vi "DblMonoPMDScan.vi"() -> ()   [LabVIEW 2009]
uses:
  <vilib>/Utility/file.llb/Write To Spreadsheet File (DBL).vi
  <vilib>/Analysis/NI_AALBase.lvlib
panel:
  in  "On":bool=TRUE
  out "Power":cluster{dbl[], dbl[]}(graph)
  out "Waveform Chart":dbl(graph)
  in  "Save":bool=TRUE
  in  "Scan Save Path":path
  in  "Exit":bool
  in  "STOP":bool
  in  "Step Time (sec)":dbl=1.0 min=0.001 max=300.0 step=0.001 format="%.3f"
  in  "Step Size (nm)":dbl=1.0 min=0.1 max=100.0 step=0.1 format="%.1f"
  in  "End":dbl=800.0 min=0.0 max=2000.0 step=0.1 format="%.1f"
  in  "Start":dbl=400.0 min=0.0 max=2000.0 step=0.1 format="%.1f"
  in  "Scan":bool
  in  "Up":bool=TRUE caption="Down"
  in  "Increment (nm)":dbl=10.0 min=0.1 max=2000.0 step=0.1 format="%.1f"
  in  "PMD Settings":T1={"Beam Diameter (mm)"=4.0, "BWIn"=0, "Averaging Rate"=300, "Auto Range"=TRUE} {"Averaging Rate" min=33 max=5000 step=1; "BWIn" items=["HIGH", "LOW"]; "Beam Diameter (mm)" min=1.0 max=9.0 step=0.5}
  in  "Step":bool
  out "Busy":bool
  in  "Send Command":bool
  in  "Command":u16(ring) items=["nm", "goto", "nm/min", "VIS grating", "IR grating"]
  in  "Wavelength (nm)":dbl=100.0 min=0.0 max=2000.0 step=0.1 format="%.1f"
  in  "Scan Speed (nm/min)":dbl=100.0 min=1.0 max=500.0 step=0.1 format="%.1f"
  out "Done?":string
  in  "Send Question":bool
  in  "Ask?":u16(ring) items=["?nm", "?nm/min", "?grating", "?turret", "?gratings"]
  out "Power (W)":dbl format="%^#_9e"
  in  "Zero?":bool
  out "PM Error log":string
  out "AUTO?":bool
  out "Zero Value":dbl format="%#.3p"
  out "Rng":string
  in  "Range":i16=1 min=1 max=6 step=1
  in  "Mono Port":refnum<visa-resource-name>="COM5"
  out "IDN String":string
  out "Sensor SN":string
  out "Sensor Name":string
  out "Reply":string caption="Mono Response"
  # "Range Settings"
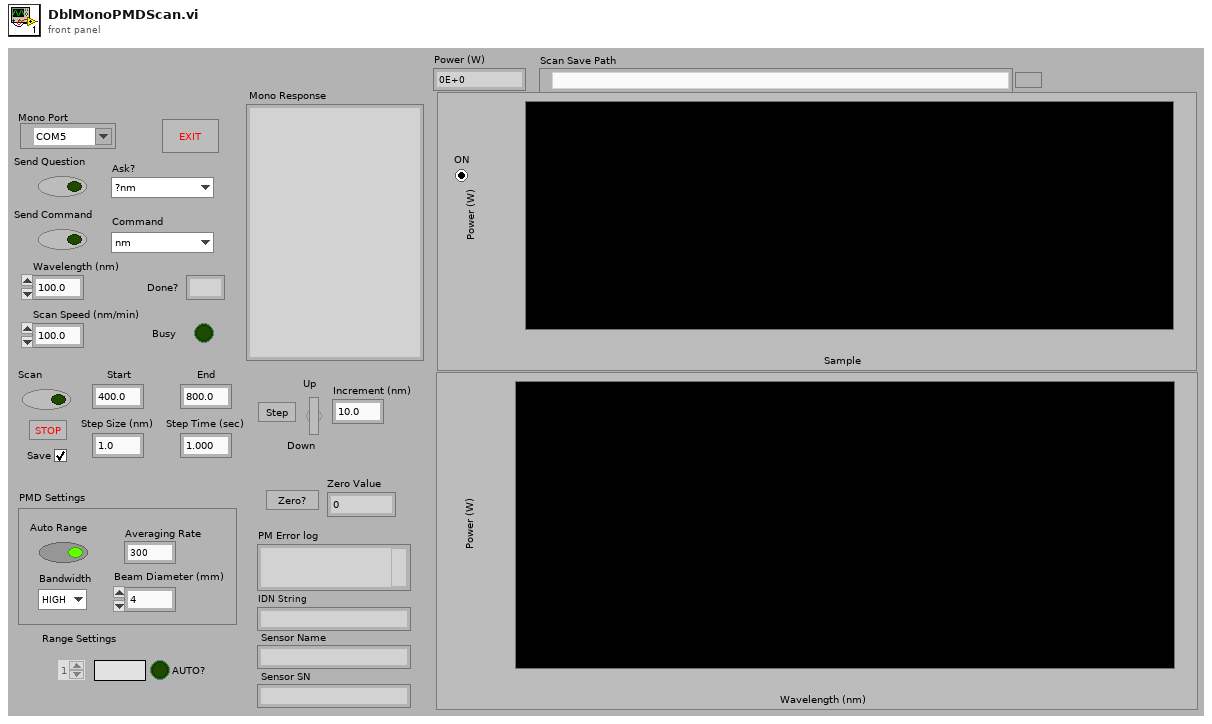
[diagram p1: front panel]
types:
  T1 = cluster{"Beam Diameter (mm)":dbl, "BWIn":u16, "Averaging Rate":i32, "Auto Range":bool}
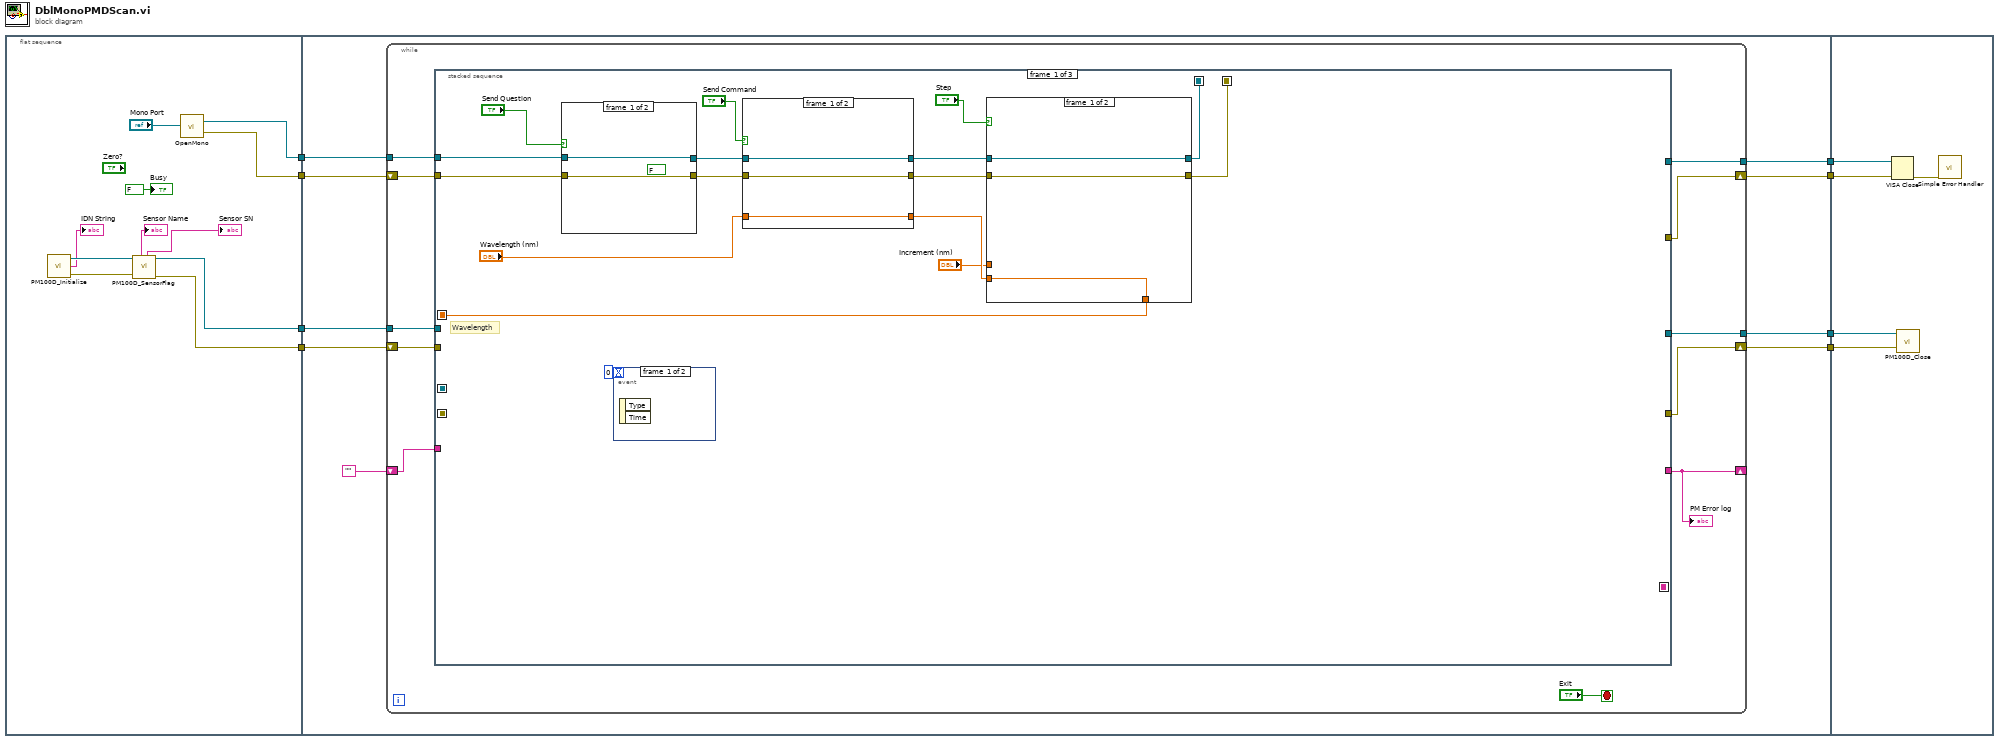
[diagram p0: block diagram]
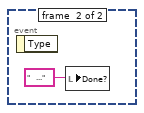
[diagram p2: hidden frame]
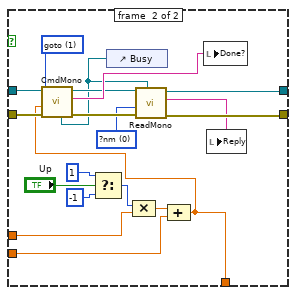
[diagram p3: hidden frame]
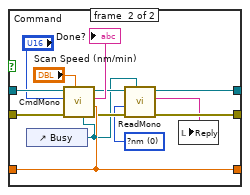
[diagram p4: hidden frame]
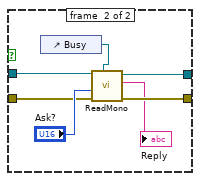
[diagram p5: hidden frame]
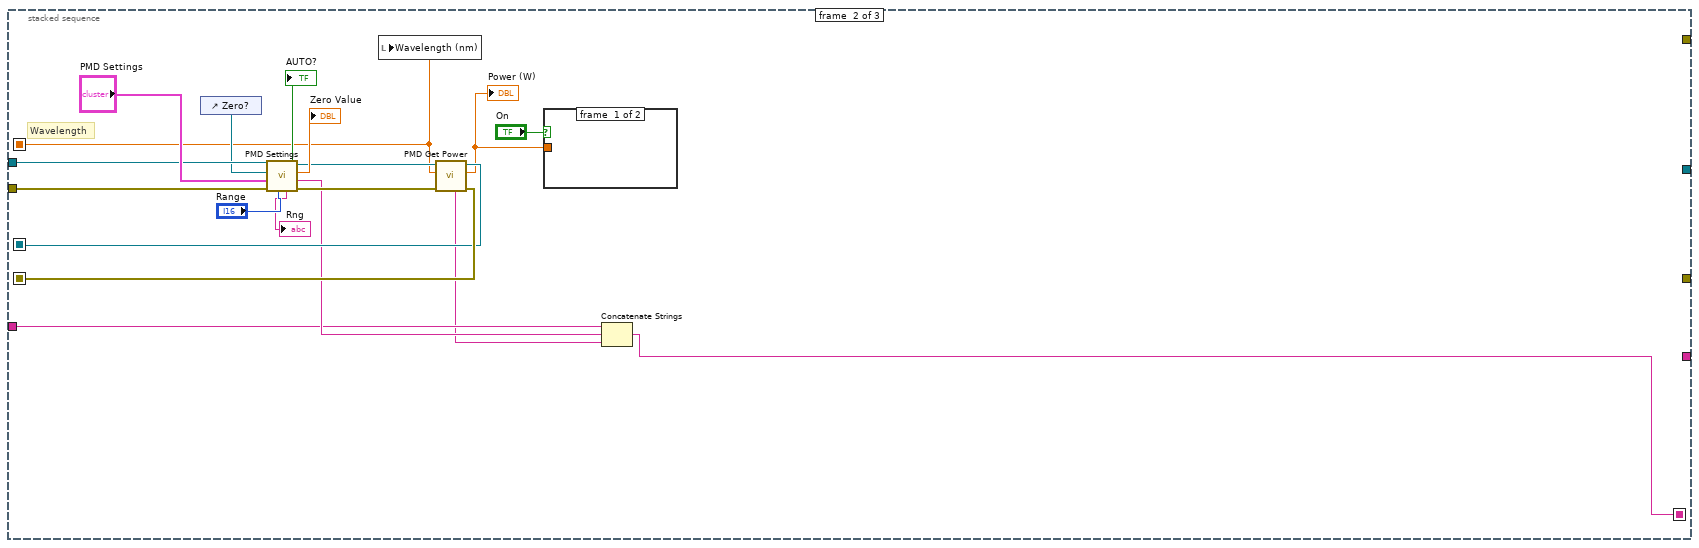
[diagram p6: hidden frame]
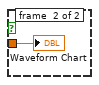
[diagram p7: hidden frame]
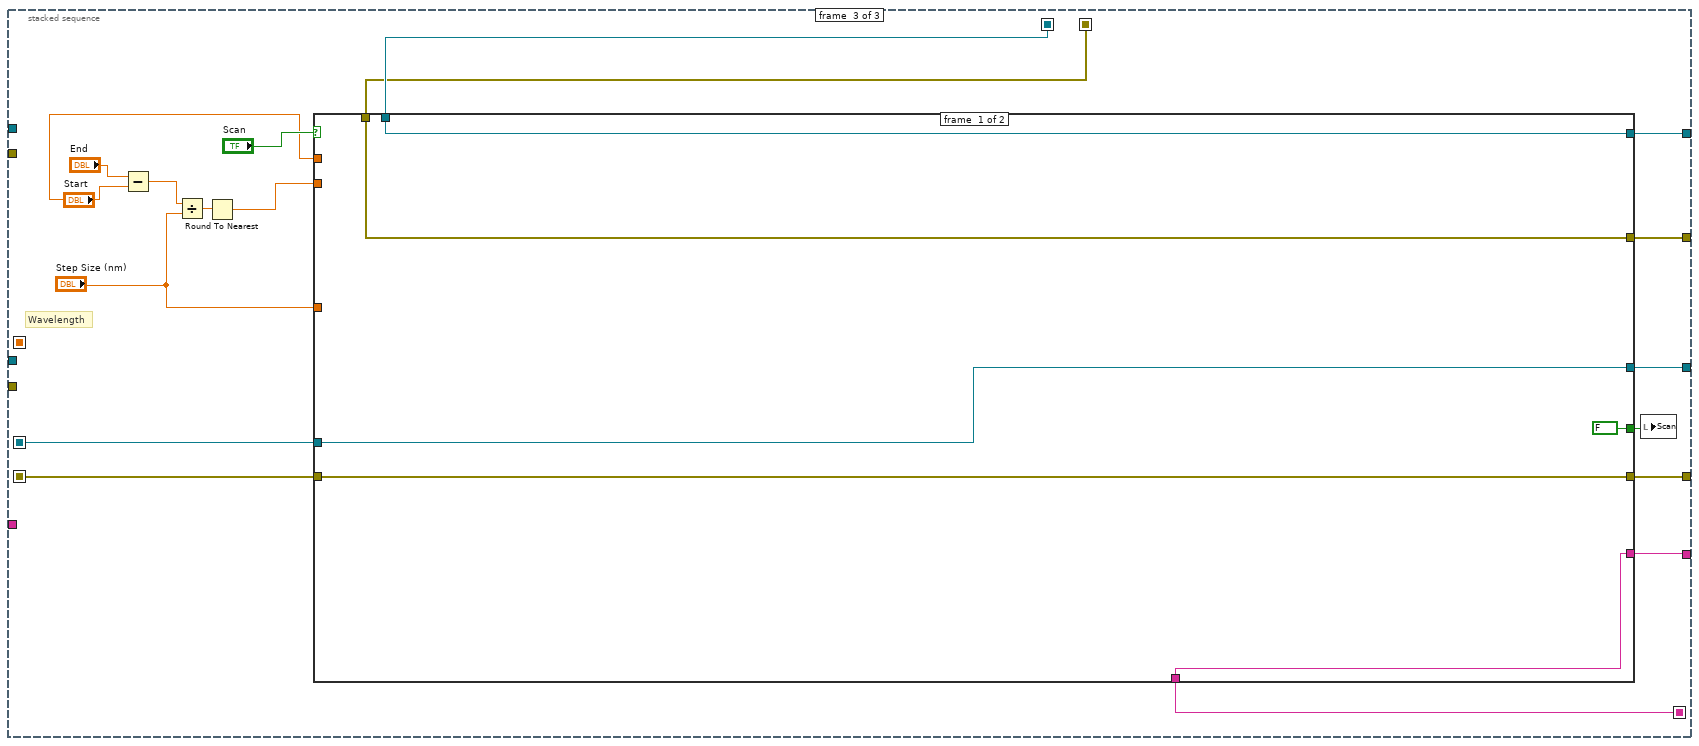
[diagram p8: hidden frame]
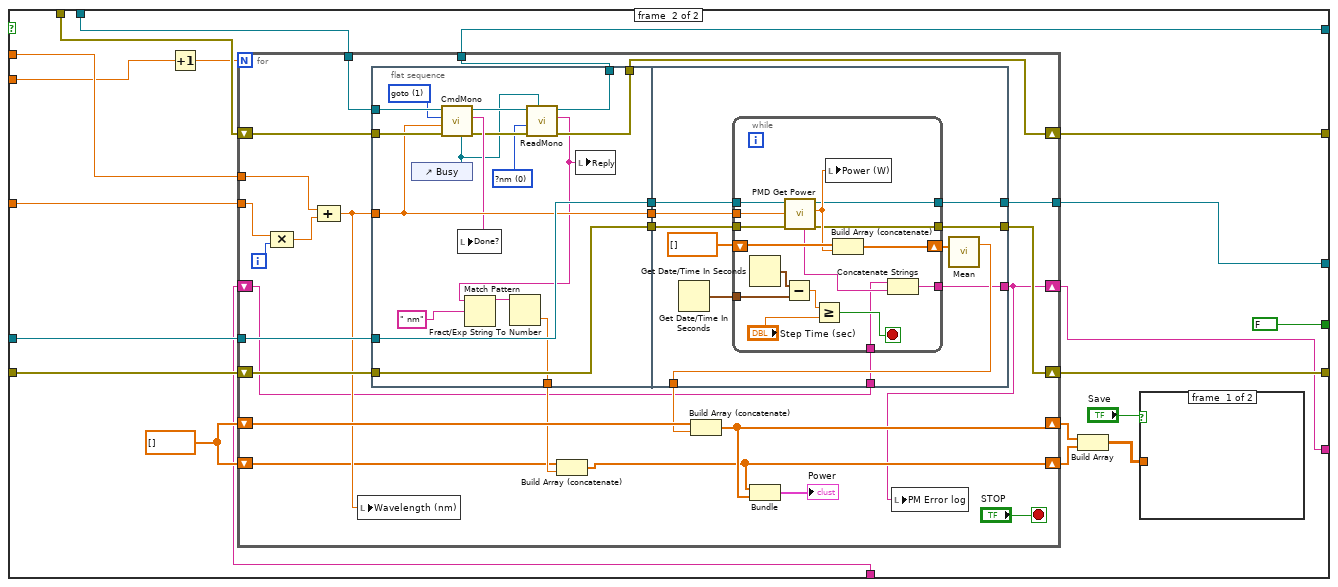
[diagram p9: hidden frame]
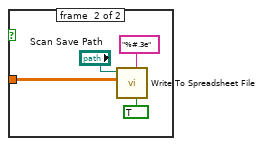
[diagram p10: hidden frame]
diagram:
  n1 = flat-sequence {
    tunnel: [w14] -> w8
    tunnel: [w13] -> w7
    tunnel: [w12] -> w6
    tunnel: [w11] -> w5
    tunnel: w8 -> [w27]
    tunnel: w7 -> [w28]
    tunnel: w6 -> [w26]
    tunnel: w5 -> [w25]
    tunnel: [w24] -> w4
    tunnel: [w23] -> w3
    tunnel: [w22] -> w2
    tunnel: [w21] -> w1
    tunnel: w4 -> [w245]
    tunnel: w3 -> [w244]
    tunnel: w2 -> [w243]
    tunnel: w1 -> [w242]
    frame #0 {
      n2 = call "PM100D_Initialize.vi"() -> ("error out"=w18:errorcluster, "Instrument"=→"IDN String":string, "VISA out"=w19:refnum<visa-resource-name>)  [unwired: 2 in, 1 out]
      n3 = call "PM100D_SensorFlag.vi"("error in (no error)"=w18, "VISA in"=w19) -> ("error out"=w14:errorcluster, "VISA out"=w13:refnum<visa-resource-name>, "sn"=→"Sensor SN":string, "name"=→"Sensor Name":string)  [unwired: 2 in, 4 out]
      n4 = call "OpenMono.vi"("Mono Port"="Mono Port") -> ("VISA resource name out"=w12:refnum<visa-resource-name>, "error out"=w11:errorcluster)
      "Busy" <- FALSE ("Busy")
    }
    frame #1 {
      n5 = while {
        tunnel: w28 -> [w37]
        tunnel: w26 -> [w39]
        tunnel: [w34] -> w23
        tunnel: [w32] -> w21
        shift-right: [w31] -> w22
        shift-left: w27 -> [w36]
        shift-right: [w33] -> w24
        shift-left: w25 -> [w38]
        shift-right: [w29] -> _
        shift-left: "" -> [w30]
        stop <- "Exit" stop-if-true
        n6 = stacked-sequence {
          seq-local: [w40 _ _] -> [_ w104 _]
          seq-local: [w45 _ _] -> [_ _ w134]
          seq-local: [w44 _ _] -> [_ _ w133]
          seq-local: [_ w112 _] -> [_ _ w132]
          seq-local: [_ w113 _] -> [_ _ w131]
          seq-local: [_ w105 _] -> [_ _ w125]
          tunnel: w39 -> [w51 _ _]
          tunnel: w38 -> [w50 _ _]
          tunnel: w37 -> [_ w115 _]
          tunnel: w36 -> [_ w114 _]
          tunnel: [_ _ w130] -> w34
          tunnel: [_ _ w129] -> w33
          tunnel: [_ _ w128] -> w32
          tunnel: [_ _ w127] -> w31
          tunnel: w30 -> [_ w107 _]
          tunnel: [_ _ w124] -> w29
          frame #0 {
            # "Wavelength"
            n7 = case shown="True" "Send Question" {
              tunnel: w51 -> [w96 w102]
              tunnel: w50 -> [w95 w101]
              tunnel: [w96 w100] -> w53
              tunnel: [w95 w99] -> w52
              frame #0 {
                (unwired) FALSE ("Read Error")
              }
              frame #1 {
                n8 = control-ref of="Busy"() -> (w97:refnum<vi>)
                n9 = call "ReadMono.vi"("Busy"=w97, "error in (no error)"=w101, "Cmd"="Ask?", "Mono Port"=w102) -> ("error out"=w99:errorcluster, "Response"=→"Reply":string, "Mono Port Out"=w100:refnum<visa-resource-name>)  [unwired: 2 in, 1 out]
              }
            }
            n10 = event shown="[1] \"Send Command\", \"Step\": Mouse Up" {
              selector: _ -> [_ _]
              dyn-events: _ -> [_ _]
              timeout: 0 -> [_ _]
              event #0 {
                n11 = event-data() -> ()  [unwired: 1 in, 2 out]
              }
              event #1 {
                n12 = event-data() -> ()  [unwired: 1 in, 1 out]
                n13 = local write "Done?"("   ..." ("Done?")) -> ()
              }
            }
            n14 = case shown="True" "Send Command" {
              tunnel: w53 -> [w81 w94]
              tunnel: w52 -> [w80 w93]
              tunnel: [w81 w86] -> w48
              tunnel: [w80 w85] -> w47
              tunnel: "Wavelength (nm)" -> [w79 w89]
              tunnel: [w79 w89] -> w46
              frame #0 {
              }
              frame #1 {
                w84 = u16 0 items=["?nm", "?nm/min", "?grating", "?turret", "?gratings"] ("Cmd")
                n15 = control-ref of="Busy"() -> (w82:refnum<vi>)
                n16 = call "CmdMono.vi"("Busy"=w82, "Scan Speed (nm/min)"="Scan Speed (nm/min)", "error in (no error)"=w93, "Wavelength (nm)"=w89, "Cmd"="Command", "Mono Port"=w94) -> ("error out"=w87:errorcluster, "Response"=→"Done?":string, "Mono Port Out"=w88:refnum<visa-resource-name>)  [unwired: 2 in, 1 out]
                n17 = call "ReadMono.vi"("Busy"=w82, "error in (no error)"=w87, "Cmd"=w84, "Mono Port"=w88) -> ("error out"=w85:errorcluster, "Response"=w83:string, "Mono Port Out"=w86:refnum<visa-resource-name>)  [unwired: 2 in, 1 out]
                n18 = local write "Reply"(w83) -> ()
              }
            }
            n19 = case shown="True" "Step" {
              tunnel: w48 -> [w59 w78]
              tunnel: w47 -> [w58 w77]
              tunnel: w46 -> [w57 w71]
              tunnel: [w59 w64] -> w45
              tunnel: [w58 w65] -> w44
              tunnel: "Increment (nm)" -> [_ w70]
              tunnel: [w57 w60] -> w40
              frame #0 {
              }
              frame #1 {
                w62 = u16 0 items=["?nm", "?nm/min", "?grating", "?turret", "?gratings"] ("Cmd")
                w69 = u16 1 items=["nm", "goto", "nm/min", "VIS grating", "IR grating"] ("Cmd")
                n20 = Select(t=1, s="Up", f=-1) -> (s? t:f=w76:i32)
                n21 = control-ref of="Busy"() -> (w61:refnum<vi>)
                n22 = Compound Arithmetic op=MULTIPLY(w76, w70) -> (w72:dbl)
                n23 = Compound Arithmetic op=ADD(w72, w71) -> (w60:dbl)
                n24 = call "CmdMono.vi"("Busy"=w61, "error in (no error)"=w77, "Wavelength (nm)"=w60, "Cmd"=w69, "Mono Port"=w78) -> ("error out"=w66:errorcluster, "Response"=w68:string, "Mono Port Out"=w67:refnum<visa-resource-name>)  [unwired: 3 in, 1 out]
                n25 = call "ReadMono.vi"("Busy"=w61, "error in (no error)"=w66, "Cmd"=w62, "Mono Port"=w67) -> ("error out"=w65:errorcluster, "Response"=w63:string, "Mono Port Out"=w64:refnum<visa-resource-name>)  [unwired: 2 in, 1 out]
                n26 = local write "Done?"(w68) -> ()
                n27 = local write "Reply"(w63) -> ()
              }
            }
          }
          frame #1 {
            # "Wavelength"
            n28 = control-ref of="Zero?"() -> (w109:refnum<vi>)
            n29 = call "PMD Settings.vi"("Visa In"=w115, "Zero?"=w109, "PMD Settings In"="PMD Settings", "Error In"=w114, "Range"="Range") -> ("AUTO?"=→"AUTO?":bool, "Rng"=→"Rng":string, "Visa Out"=w118:refnum<visa-resource-name>, "ZeroValue"=→"Zero Value":dbl, "PM Error log"=w108:string, "error out"=w117:errorcluster)
            n30 = local write "Wavelength (nm)"(w104) -> ()
            n31 = call "PMD Get Power.vi"("VISA In"=w118, "Wavelength (nm)"=w104, "error in"=w117) -> ("PMD Error"=w106:string, "VISA out"=w112:refnum<visa-resource-name>, "Readout value"=w111:dbl, "error out"=w113:errorcluster)  [unwired: 1 in, 2 out]
            "Power (W)" <- w111
            n32 = case shown="True" "On" {
              tunnel: w111 -> [_ w123]
              frame #0 {
              }
              frame #1 {
                "Waveform Chart" <- w123
              }
            }
            n33 = Concatenate Strings(w107, w108, w106) -> (w105:string)
          }
          frame #2 {
            # "Wavelength"
            n34 = Subtract(x="End", y="Start") -> (x-y=w139:dbl)
            n35 = Divide(x=w139, y="Step Size (nm)") -> (x/y=w138:dbl)
            n36 = Round To Nearest(number=w138) -> (nearest integer value=w137:dbl)
            n37 = case shown="True" "Scan" {
              tunnel: w137 -> [_ w162]
              tunnel: w133 -> [w145 w164]
              tunnel: w134 -> [w144 w165]
              tunnel: "Start" -> [_ w167]
              tunnel: "Step Size (nm)" -> [_ w166]
              tunnel: w132 -> [w147 w160]
              tunnel: w131 -> [w146 w159]
              tunnel: [w147 w157] -> w128
              tunnel: [w146 w158] -> w127
              tunnel: [w145 w156] -> w129
              tunnel: [w144 w155] -> w130
              tunnel: [FALSE ("Scan") FALSE ("Scan")] -> w126
              tunnel: w125 -> [w142 w149]
              tunnel: [w142 w148] -> w124
              frame #0 {
              }
              frame #1 {
                w163 = dbl[] []
                n38 = Increment(x=w162) -> (x+1=w161:dbl)
                n39 = for {
                  N: w161 -> [_]
                  tunnel: w165 -> [w194]
                  tunnel: w167 -> [w190]
                  tunnel: w166 -> [w192]
                  shift-right: [w178] -> w154
                  shift-left: w163 -> [w197]
                  shift-right: [w189] -> w156
                  shift-left: w164 -> [w195]
                  shift-right: [w174] -> w153
                  shift-left: w163 -> [w175]
                  tunnel: w160 -> [w187]
                  shift-right: [w182] -> w158
                  shift-left: w159 -> [w186]
                  tunnel: [w181] -> w157
                  tunnel: [w180] -> w155
                  shift-right: [w172] -> w148
                  shift-left: w149 -> [w173]
                  i -> [w193]
                  stop <- "STOP" stop-if-true
                  n40 = Compound Arithmetic op=MULTIPLY(w192, w193) -> (w191:dbl)
                  n41 = Compound Arithmetic op=ADD(w190, w191) -> (w177:dbl)
                  n42 = local write "Wavelength (nm)"(w177) -> ()
                  n43 = flat-sequence {
                    tunnel: w195 -> [w214]
                    tunnel: w194 -> [w213]
                    tunnel: w177 -> [w209]
                    tunnel: [w202] -> w189
                    tunnel: w187 -> [w211]
                    tunnel: w186 -> [w210]
                    tunnel: [w211] -> w185
                    tunnel: [w210] -> w184
                    tunnel: [w209] -> w183
                    tunnel: [w203] -> w180
                    tunnel: [w198] -> w176
                    tunnel: [w222] -> w196
                    tunnel: w185 -> [w221]
                    tunnel: w184 -> [w220]
                    tunnel: w183 -> [w219]
                    tunnel: [w218] -> w182
                    tunnel: [w217] -> w181
                    tunnel: w173 -> [w216]
                    tunnel: [w215] -> w172
                    frame #0 {
                      w205 = u16 0 items=["?nm", "?nm/min", "?grating", "?turret", "?gratings"] ("Cmd")
                      w212 = u16 1 items=["nm", "goto", "nm/min", "VIS grating", "IR grating"] ("Cmd")
                      n44 = control-ref of="Busy"() -> (w204:refnum<vi>)
                      n45 = call "CmdMono.vi"("Busy"=w204, "error in (no error)"=w214, "Wavelength (nm)"=w209, "Cmd"=w212, "Mono Port"=w213) -> ("error out"=w206:errorcluster, "Response"=w208:string, "Mono Port Out"=w207:refnum<visa-resource-name>)  [unwired: 3 in, 1 out]
                      n46 = local write "Done?"(w208) -> ()
                      n47 = call "ReadMono.vi"("Busy"=w204, "error in (no error)"=w206, "Cmd"=w205, "Mono Port"=w207) -> ("error out"=w202:errorcluster, "Response"=w200:string, "Mono Port Out"=w203:refnum<visa-resource-name>)  [unwired: 2 in, 1 out]
                      n48 = Match Pattern(string=w200, regular expression=" nm") -> (before substring=w199:string)  [unwired: 1 in, 3 out]
                      n49 = Fract/Exp String To Number(string=w199) -> (number=w198:dbl)  [unwired: 3 in, 1 out]
                      n50 = local write "Reply"(w200) -> ()
                    }
                    frame #1 {
                      n51 = Get Date/Time In Seconds() -> (seconds since 1Jan1904=w224:timestamp)
                      n52 = while {
                        shift-right: [w240] -> w223
                        shift-left: dbl[] [] -> [w241]
                        tunnel: w224 -> [w238]
                        tunnel: w221 -> [w233]
                        tunnel: w220 -> [w232]
                        tunnel: w219 -> [w231]
                        tunnel: [w230] -> w218
                        tunnel: [w229] -> w217
                        tunnel: w216 -> [w227]
                        tunnel: [w226] -> w215
                        stop <- w235 stop-if-true
                        n53 = Get Date/Time In Seconds() -> (seconds since 1Jan1904=w239:timestamp)
                        n54 = Subtract(x=w239, y=w238) -> (x-y=w237:dbl)
                        n55 = call "PMD Get Power.vi"("VISA In"=w233, "Wavelength (nm)"=w231, "error in"=w232) -> ("PMD Error"=w228:string, "VISA out"=w229:refnum<visa-resource-name>, "Readout value"=w234:dbl, "error out"=w230:errorcluster)  [unwired: 1 in, 2 out]
                        n56 = Greater Or Equal?(x=w237, y="Step Time (sec)") -> (x >= y?=w235:bool)
                        n57 = local write "Power (W)"(w234) -> ()
                        n58 = Build Array (concatenate)(w241, w234) -> (w240:dbl[])
                        n59 = Concatenate Strings(w227, w228) -> (w226:string)
                      }
                      n60 = call <vilib>:"Mean.vi"("X"=w223) -> ("mean"=w222:dbl)  [unwired: 1 out]
                    }
                  }
                  n61 = Build Array (concatenate)(w175, w176) -> (w174:dbl[])
                  n62 = Build Array (concatenate)(w197, w196) -> (w178:dbl[])
                  n63 = Bundle(w174, w178) -> (→"Power":cluster{dbl[], dbl[]})  [unwired: 1 in]
                  n64 = local write "PM Error log"(w172) -> ()
                }
                n65 = Build Array(w154, w153) -> (w152:dbl[][])
                n66 = case shown="True" "Save" {
                  tunnel: w152 -> [_ w168]
                  frame #0 {
                  }
                  frame #1 {
                    n67 = call-poly <vilib>:"Write To Spreadsheet File.vi"("transpose? (no:F)"=TRUE, "format (%.3f)"="%#.3e", "2D data"=w168, "file path (dialog if empty)"="Scan Save Path") -> ()  [unwired: 4 in, 1 out]
                  }
                }
              }
            }
            n68 = local write "Scan"(w126) -> ()
          }
        }
        "PM Error log" <- w29
      }
    }
    frame #2 {
      n69 = VISA Close(VISA resource name=w244, error in (no error)=w245) -> (error out=w246:errorcluster)
      n70 = call "PM100D_Close.vi"("error in (no error)"=w243, "VISA resource name"=w242) -> ()  [unwired: 2 in]
      n71 = call <vilib>:"Simple Error Handler.vi"("error in (no error)"=w246) -> ()  [unwired: 1 in, 8 out]
    }
  }
